vi "S2C_FORNAX_Proc_VersionCmdMsg.vi"(8 "Error In":errorcluster, 10 "Cmd In":string, 11 "JSON In":string) -> (0 "Error Out":errorcluster, 2 "Cmd Out":string, 3 "JSON Out":string)   [LabVIEW 2015]
uses:
  S2C_FORNAX_Proc_Globals.vi
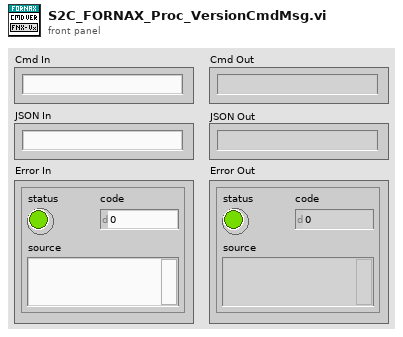
[diagram p1: front panel]
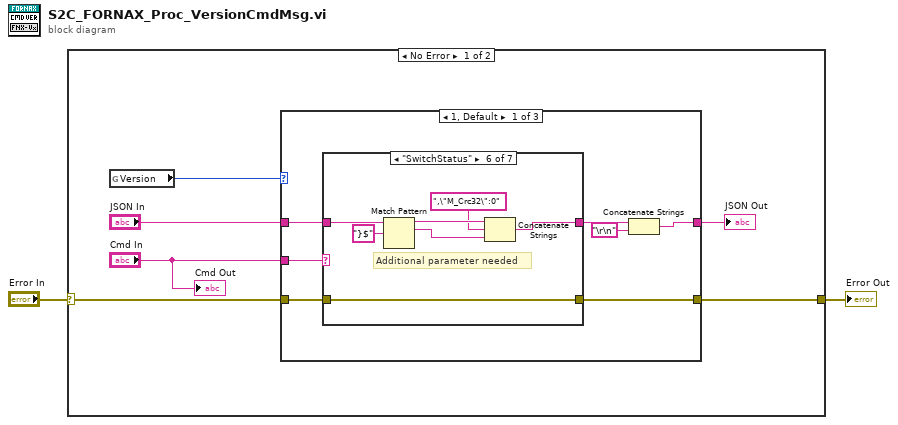
[diagram p0: block diagram]
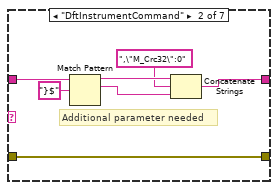
[diagram p3: hidden frame]
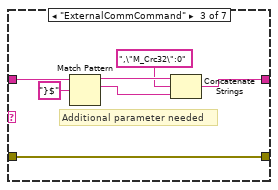
[diagram p4: hidden frame]
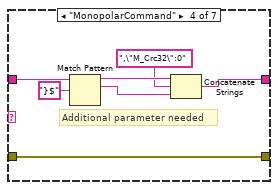
[diagram p5: hidden frame]
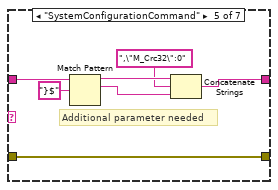
[diagram p6: hidden frame]
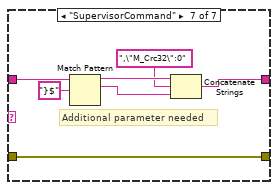
[diagram p7: hidden frame]
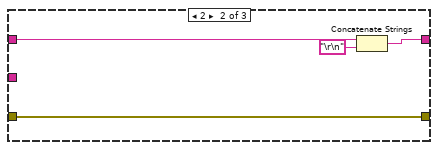
[diagram p8: hidden frame]
diagram:
  n1 = case shown="No Error" "Error In" {
    selector: "Error In" -> [w8 w66]
    tunnel: [w6 w66] -> w1
    frame No Error {
      n2 = global read "S2C_FORNAX_Proc_Globals.vi" "Version"() -> (w7:i32)
      n3 = case shown="1, Default" w7 {
        tunnel: w8 -> [w15 w61 w65]
        tunnel: [w14 w61 w65] -> w6
        tunnel: "Cmd In" -> [w13 _ _]
        tunnel: [w10 w63 w64] -> w5
        tunnel: "JSON In" -> [w12 w60 w64]
        frame 1, Default {
          n4 = case shown="\"SwitchStatus\"" w13 {
            tunnel: w15 -> [w17 w20 w27 w34 w41 w48 w55]
            tunnel: [w17 w20 w27 w34 w41 w48 w55] -> w14
            tunnel: [w16 w19 w26 w33 w40 w47 w54] -> w11
            tunnel: w12 -> [w16 w18 w25 w32 w39 w46 w53]
            frame "Other", Default {
            }
            frame "DftInstrumentCommand" {
              # "Additional parameter needed"
              n5 = Match Pattern(string=w18, regular expression="}$") -> (before substring=w23:string, match substring=w21:string)  [unwired: 1 in, 2 out]
              n6 = Concatenate Strings(w23, ",\"M_Crc32\":0", w21) -> (w19:string)
            }
            frame "ExternalCommCommand" {
              # "Additional parameter needed"
              n7 = Match Pattern(string=w25, regular expression="}$") -> (before substring=w30:string, match substring=w28:string)  [unwired: 1 in, 2 out]
              n8 = Concatenate Strings(w30, ",\"M_Crc32\":0", w28) -> (w26:string)
            }
            frame "MonopolarCommand" {
              # "Additional parameter needed"
              n9 = Match Pattern(string=w32, regular expression="}$") -> (before substring=w37:string, match substring=w35:string)  [unwired: 1 in, 2 out]
              n10 = Concatenate Strings(w37, ",\"M_Crc32\":0", w35) -> (w33:string)
            }
            frame "SystemConfigurationCommand" {
              # "Additional parameter needed"
              n11 = Match Pattern(string=w39, regular expression="}$") -> (before substring=w44:string, match substring=w42:string)  [unwired: 1 in, 2 out]
              n12 = Concatenate Strings(w44, ",\"M_Crc32\":0", w42) -> (w40:string)
            }
            frame "SwitchStatus" {
              # "Additional parameter needed"
              n13 = Match Pattern(string=w46, regular expression="}$") -> (before substring=w51:string, match substring=w49:string)  [unwired: 1 in, 2 out]
              n14 = Concatenate Strings(w51, ",\"M_Crc32\":0", w49) -> (w47:string)
            }
            frame "SupervisorCommand" {
              # "Additional parameter needed"
              n15 = Match Pattern(string=w53, regular expression="}$") -> (before substring=w58:string, match substring=w56:string)  [unwired: 1 in, 2 out]
              n16 = Concatenate Strings(w58, ",\"M_Crc32\":0", w56) -> (w54:string)
            }
          }
          n17 = Concatenate Strings(w11, "\r\n") -> (w10:string)
        }
        frame 2 {
          n18 = Concatenate Strings(w60, "\r\n") -> (w63:string)
        }
        frame 3 {
        }
      }
      "JSON Out" <- w5
      "Cmd Out" <- "Cmd In"
    }
    frame Error {
    }
  }
  "Error Out" <- w1
